vi "Compute Base Speed for Voltage.vi"(8 "error in":errorcluster, 11 "Parrot in":refnum<class "Parrot.lvclass">) -> (0 "error out":errorcluster, 2 "Adjusted Base Speed":dbl, 3 "Parrot out":refnum<class "Parrot.lvclass">)   [LabVIEW 2020, in "Parrot.lvclass"]
uses:
  Parrot.lvclass
  Parrot.lvclass/Parrot.ctl
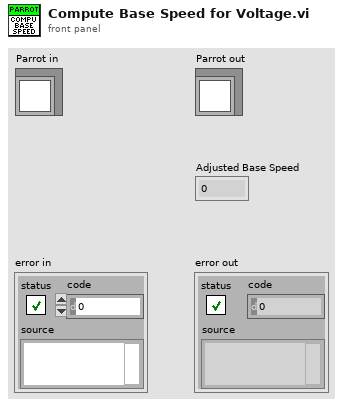
[diagram p1: front panel]
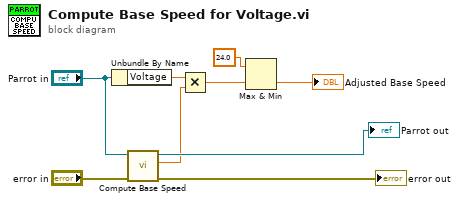
[diagram p0: block diagram]
diagram:
  n1 = Unbundle By Name("Parrot in") -> ("Voltage"=w2:dbl)
  n2 = call "Compute Base Speed.vi"("error in"="error in", "Parrot in"="Parrot in") -> ("error out"=→"error out":errorcluster, "Base Speed"=w5:dbl, "Parrot out"=→"Parrot out":refnum<class "Parrot.lvclass">)  [unwired: 7 in]
  n3 = Multiply(x=w2, y=w5) -> (x*y=w4:dbl)
  n4 = Max & Min(x=24.0, y=w4) -> (min(x,y)=→"Adjusted Base Speed":dbl)  [unwired: 1 out]
